vi "ActOnTrigOff.vi"(0 "ActionLvDialog in":refnum<class "ActionBeep.lvclass">, 1 "Data":variant, 5 "error in (no error)":errorcluster) -> (14 "ActionLvDialog out":refnum<class "ActionBeep.lvclass">, 19 "error out":errorcluster)   [LabVIEW 2017, in "ActionBeep.lvclass"]
doc: "Base class implementation (empty)."
uses:
  ActionBeep.lvclass
  <vilib>/measure/NI_MABase.lvlib
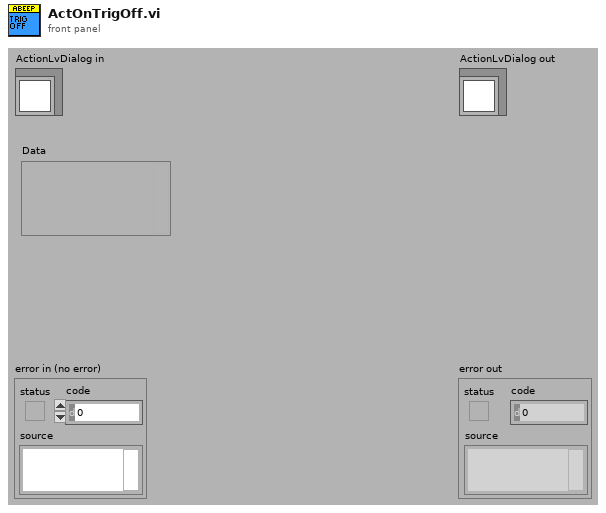
[diagram p1: front panel]
types:
  T1 = enum16{"Sine Wave", "Triangle Wave", "Square Wave", "Sawtooth Wave"}
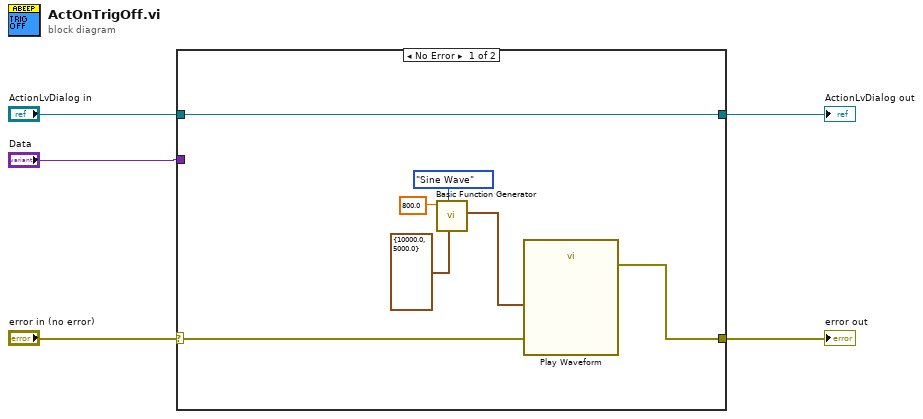
[diagram p0: block diagram]
diagram:
  n1 = case shown="No Error" "error in (no error)" {
    selector: "error in (no error)" -> [w7 w13]
    tunnel: "ActionLvDialog in" -> [w12 w14]
    tunnel: [w12 w14] -> w4
    tunnel: [w6 w13] -> w2
    tunnel: "Data" -> [_ _]
    frame No Error {
      n2 = call <vilib>:"Basic Function Generator.vi"("sampling info"=cluster{"Fs":dbl, "#s":dbl} {"Fs"=10000.0, "#s"=5000.0}, "signal type"=T1."Sine Wave", "frequency"=800.0 ("frequency (Hz)")) -> ("signal out"=w8:waveform(dbl))  [unwired: 6 in, 2 out]
      n3 = call "Play Waveform"("Data"=w8, "error in"=w7) -> ("error out"=w6:errorcluster)  [unwired: 17 in]
    }
    frame Error {
    }
  }
  "error out" <- w2
  "ActionLvDialog out" <- w4
